vi "Write Batch Table.vi"(8 "Error In":errorcluster, 11 "Database Full Information In":T1) -> (0 "Error Out":errorcluster, 3 "Database Full Information Out":T1)   [LabVIEW 2020]
uses:
  Data Clusters/Database Information.ctl
  <vilib>/addons/database/Connection.llb/Conn ObjectReference.ctl
  <vilib>/addons/database/NI_Database_API.lvlib
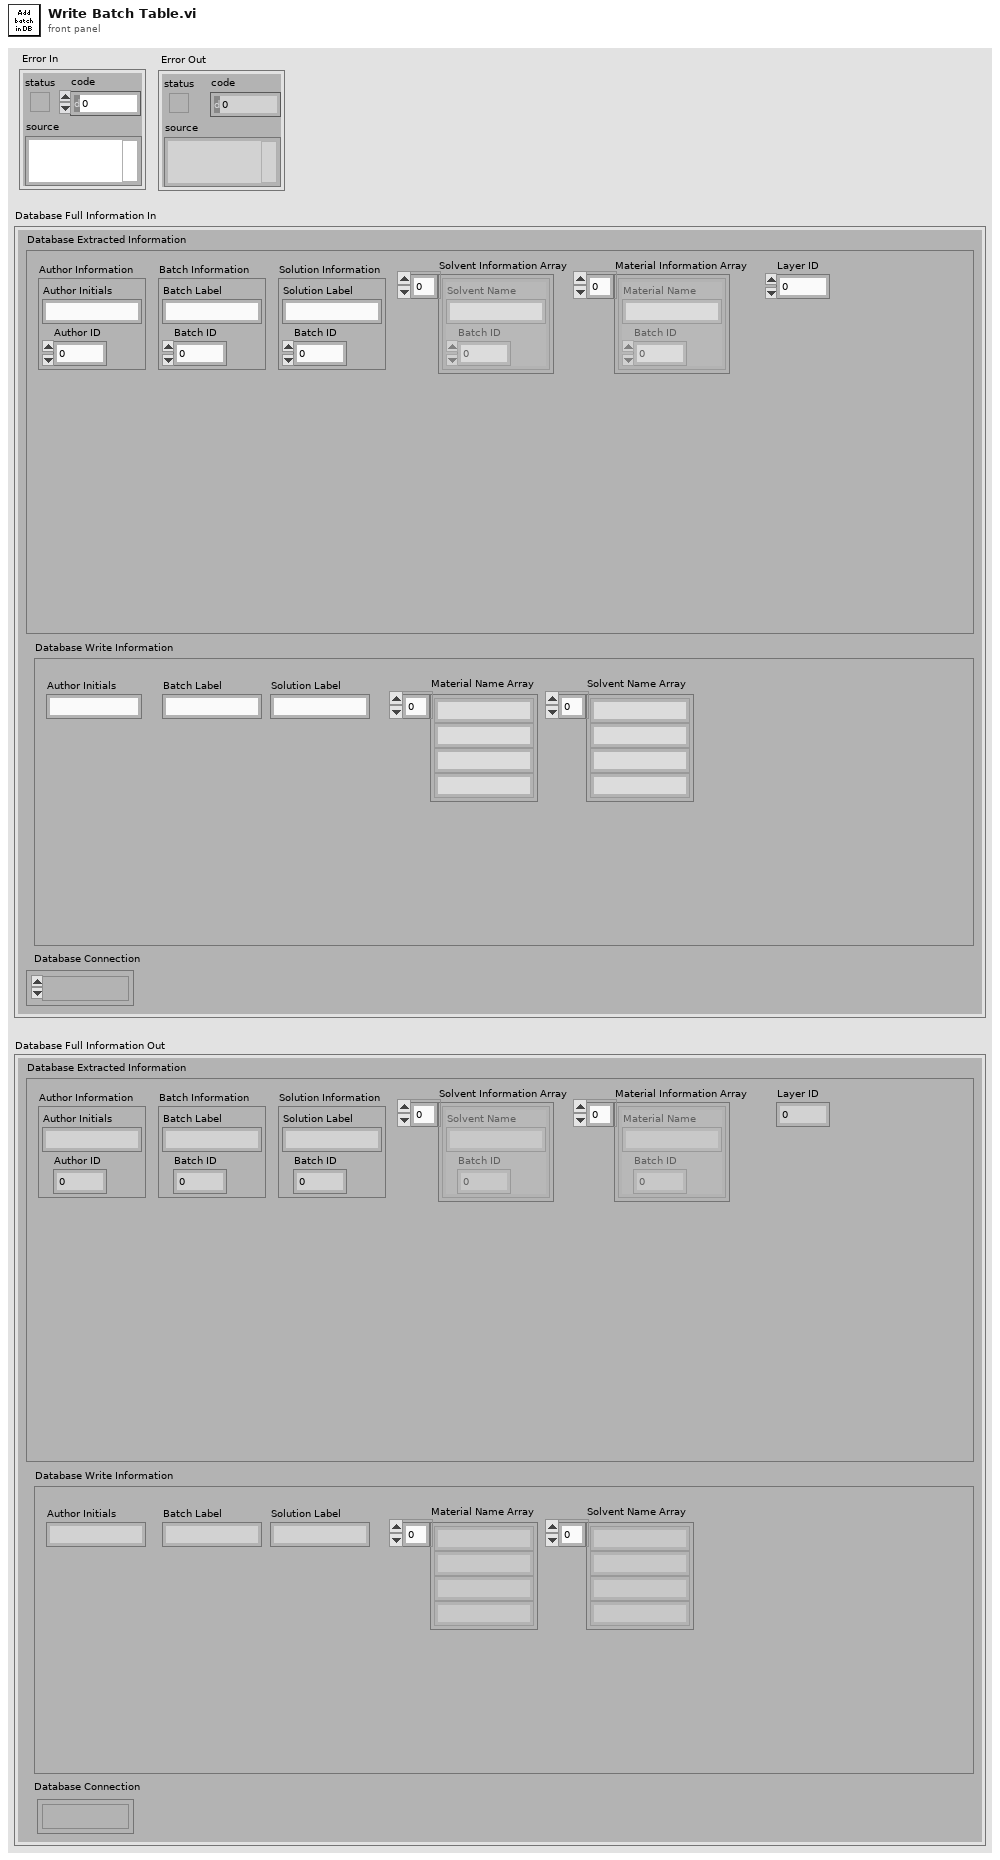
[diagram p1: front panel]
types:
  T1 = typedef "Database Information.ctl" = cluster{"Database Extracted Information":cluster{"Author Information":cluster{"Author Initials":string, "Author ID":i32}, "Batch Information":cluster{"Batch Label":string, "Batch ID":i32}, "Solution Information":cluster{"Solution Label":string, "Batch ID":i32}, "Layer ID":i32, "Solvent Information Array":cluster{"Solvent Name":string, "Batch ID":i32}[], "Material Information Array":cluster{"Material Name":string, "Batch ID":i32}[]}, "Database Write Information":cluster{"Author Initials":string, "Batch Label":string, "Solution Label":string, "Material Name Array":string[], "Solvent Name Array":string[]}, "Database Connection":T2}
  T2 = typedef "NI_Database_API.lvlib/Conn ObjectReference.ctl" = refnum<k1>
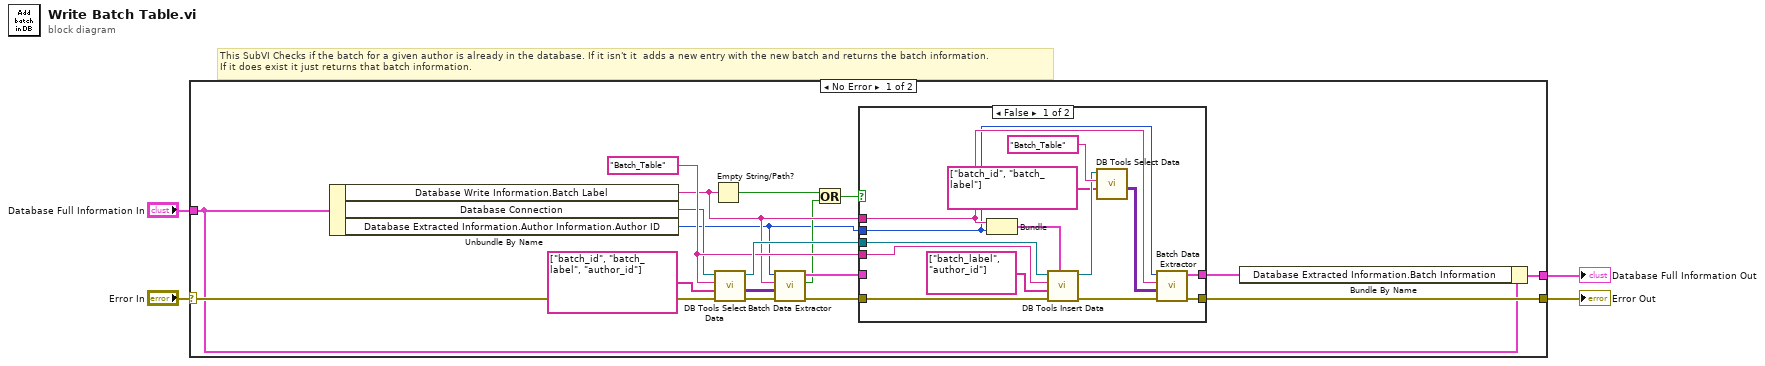
[diagram p0: block diagram]
diagram:
  # "This SubVI Checks if the batch for a given author is already in the database. If it isn't it  adds a new entry with the new batch and returns the batch information.\nIf it does exist it just returns that batch information."
  n1 = case shown="No Error" "Error In" {
    selector: "Error In" -> [w19 w40]
    tunnel: [w18 w40] -> w3
    tunnel: "Database Full Information In" -> [w7 w39]
    tunnel: [w5 w39] -> w1
    frame No Error {
      w20 = "Batch_Table" ("table")
      n2 = Unbundle By Name(w7) -> ("Database Write Information.Batch Label"=w12:string, "Database Connection"=w15:T2, "Database Extracted Information.Author Information.Author ID"=w8:i32)
      n3 = Empty String/Path?(string/path=w12) -> (empty?=w16:bool)
      n4 = call <vilib>:"DB Tools Select Data.vi"("error in (no error)"=w19, "columns"=string[] ["batch_id", "batch_label", "author_id"], "table"=w20, "connection reference"=w15) -> ("error out"=w14:errorcluster, "data"=w13:variant[][], "connection reference out"=w22:T2)  [unwired: 2 in]
      n5 = call "Batch Data Extractor.vi"("Error In"=w14, "Batch Data"=w13, "Batch Label"=w12, "Author ID"=w8) -> ("Error Out"=w9:errorcluster, "Exists?"=w10:bool, "Batch Information"=w11:cluster{"Batch Label":string, "Batch ID":i32})  [unwired: 5 in]
      n6 = Or(x=w16, y=w10) -> (x .or. y?=w17:bool)
      n7 = case shown="False" w17 {
        tunnel: w12 -> [w25 _]
        tunnel: w9 -> [w36 w38]
        tunnel: w22 -> [w35 _]
        tunnel: w20 -> [w34 _]
        tunnel: [w26 w38] -> w18
        tunnel: w11 -> [_ w37]
        tunnel: [w27 w37] -> w6
        tunnel: w8 -> [w24 _]
        frame False {
          n8 = Bundle("Batch Label"=w25, "Author ID"=w24) -> (w23:cluster{"Batch Label":string, "Author ID":i32})  [unwired: 1 in]
          n9 = call <vilib>:"DB Tools Insert Data.vi"("data"=w23, "error in (no error)"=w36, "columns"=string[] ["batch_label", "author_id"], "table"=w34, "connection reference"=w35) -> ("error out"=w29:errorcluster, "connection reference out"=w31:T2)  [unwired: 5 in]
          n10 = call <vilib>:"DB Tools Select Data.vi"("columns"=string[] ["batch_id", "batch_label"], "table"="Batch_Table", "connection reference"=w31) -> ("data"=w28:variant[][])  [unwired: 3 in, 2 out]
          n11 = call "Batch Data Extractor.vi"("Error In"=w29, "Batch Data"=w28, "Batch Label"=w25, "Author ID"=w24) -> ("Error Out"=w26:errorcluster, "Batch Information"=w27:cluster{"Batch Label":string, "Batch ID":i32})  [unwired: 5 in, 1 out]
        }
        frame True {
        }
      }
      n12 = Bundle By Name(cluster=w7, "Database Extracted Information.Batch Information"=w6) -> (w5:T1)
    }
    frame Error {
    }
  }
  "Error Out" <- w3
  "Database Full Information Out" <- w1
